vi "main.vi"() -> ()   [LabVIEW 2023] (continued)
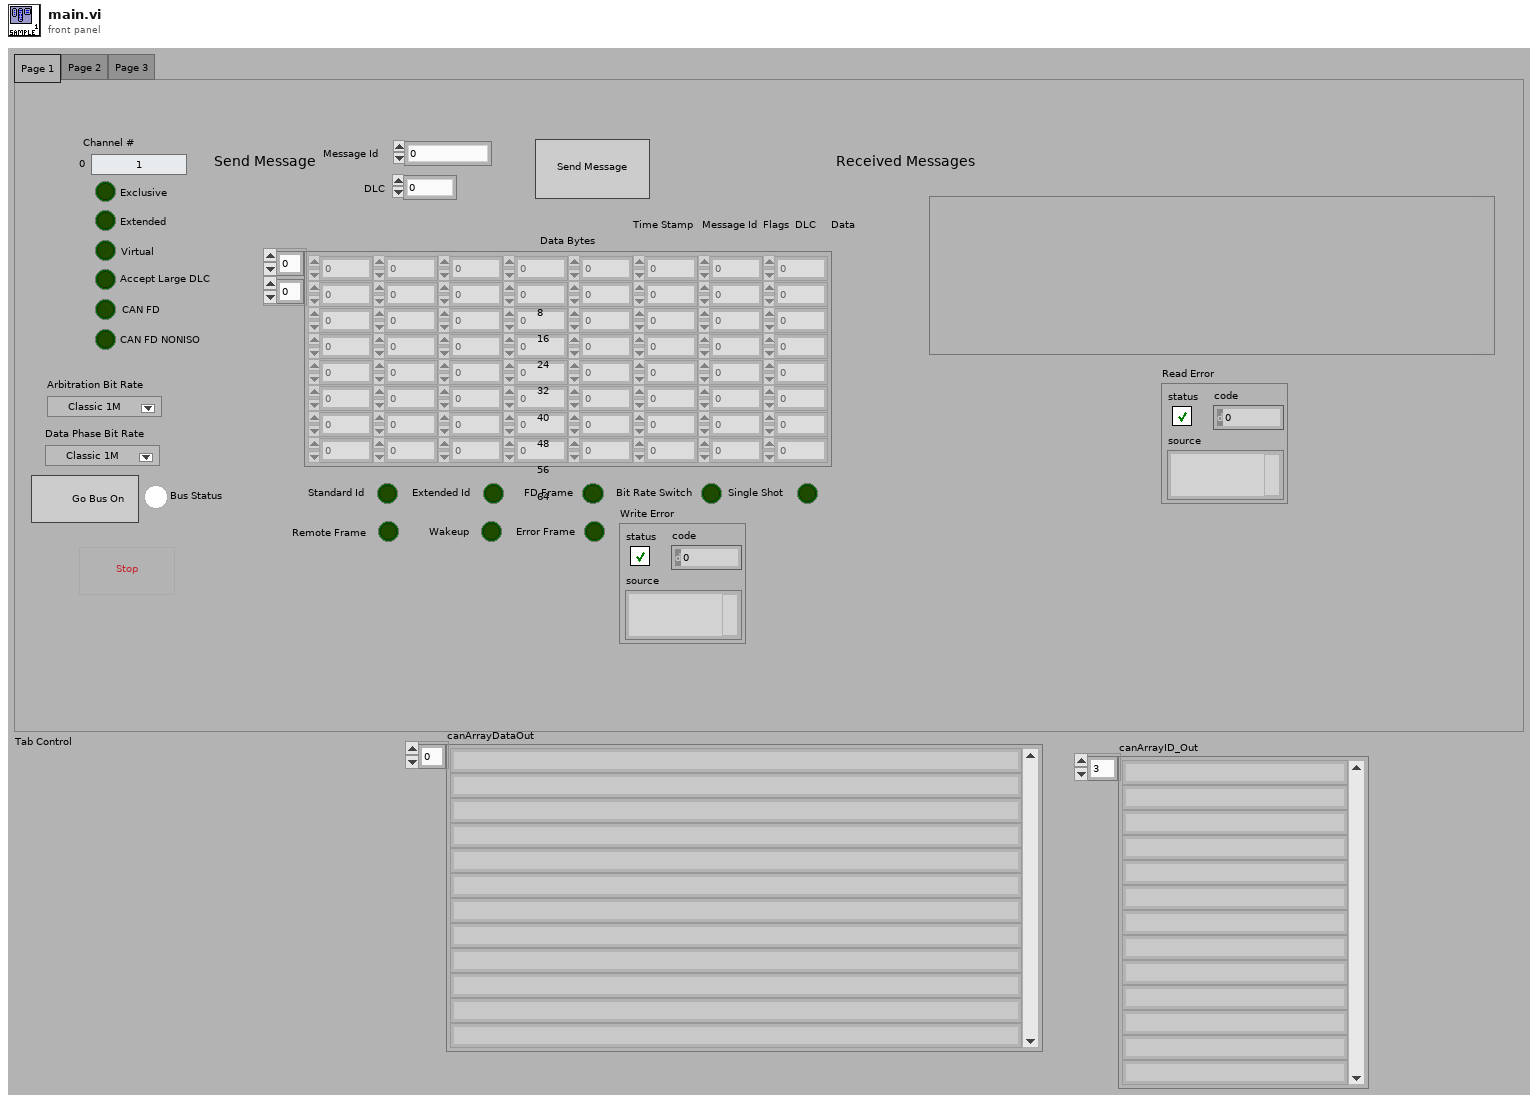
[diagram p1: front panel]
types:
  T1 = cluster{"flag 1":u32, "flag 2":u32, "flag 3":u32, "flag 4":u32}
  T2 = cluster{string, "Frame":refnum<k21>, "NameShort":string, "StartBit":u32, "NumBits":u32, "Min":dbl, "Max":dbl, "ScaleFac":dbl, "ScaleOff":dbl}[]
  T3 = typedef "readSub.ctl" = enum16{"Read", "Process"}
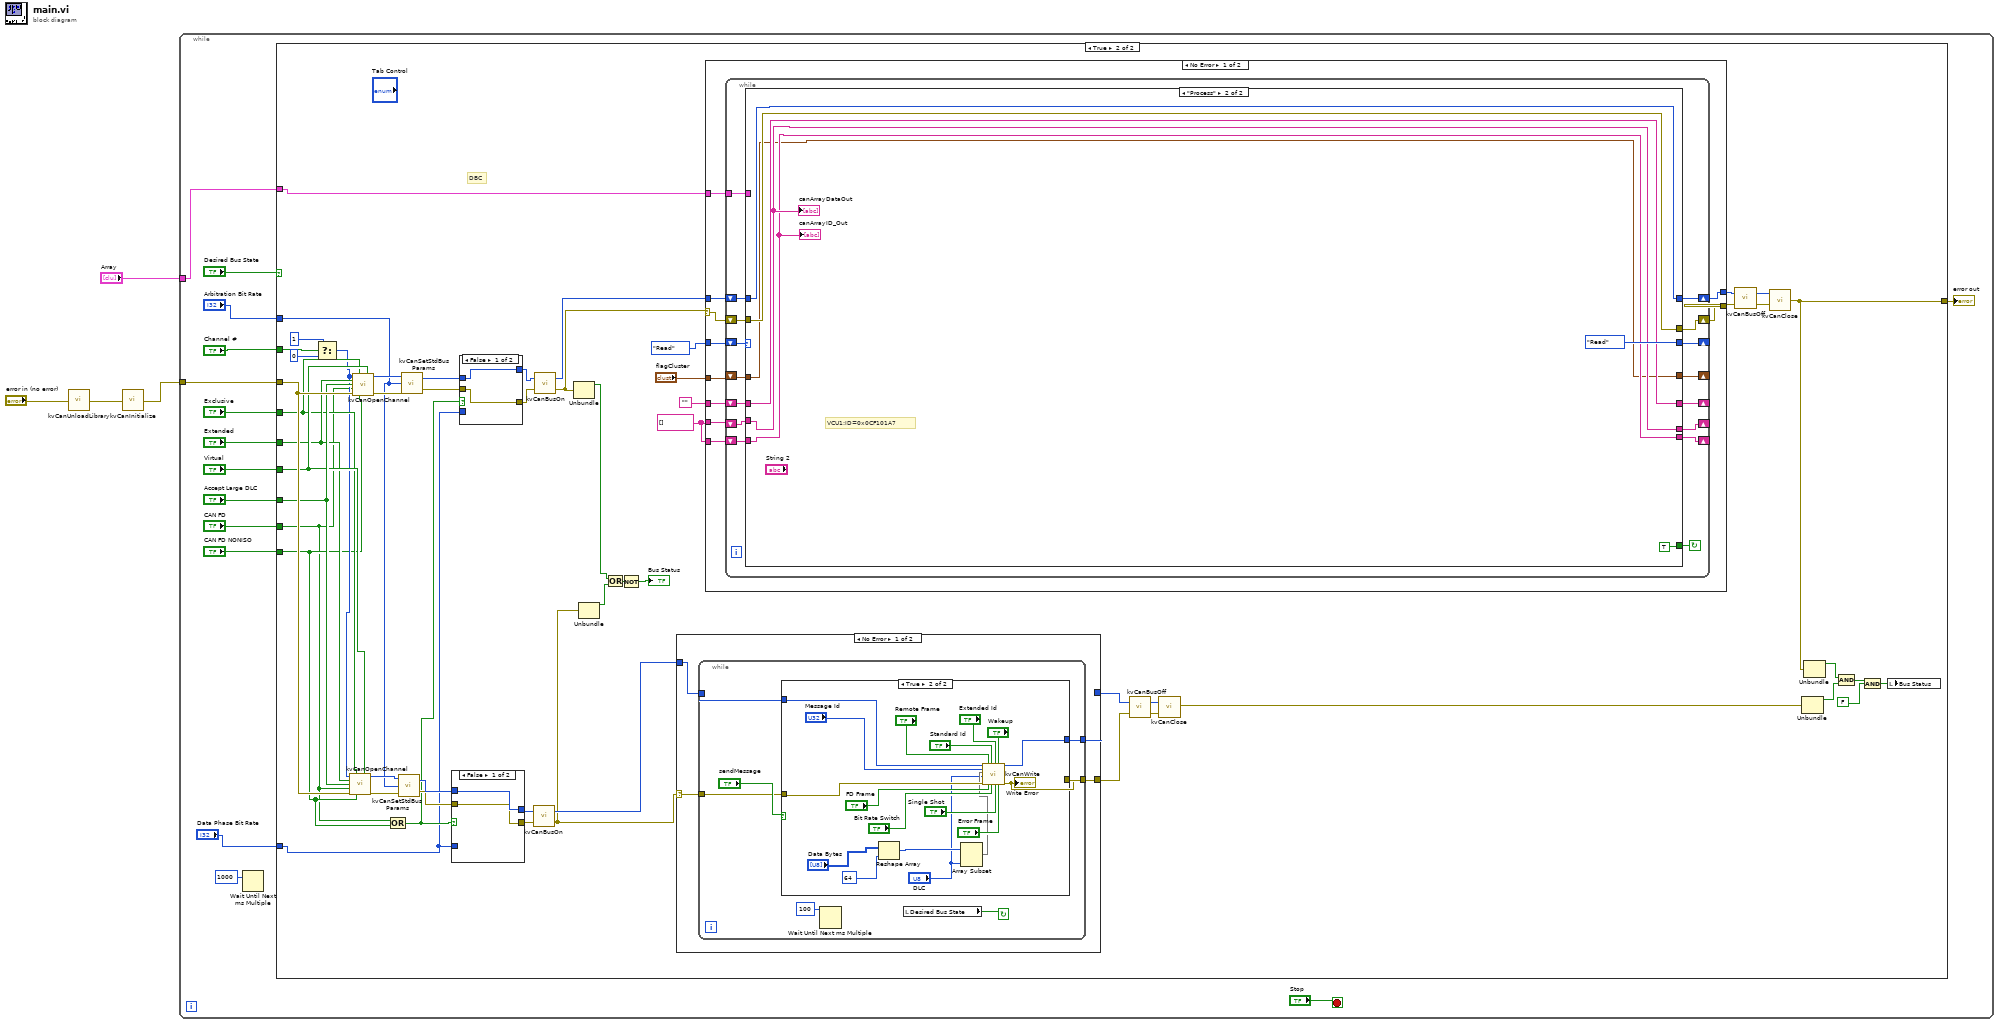
[diagram p0: block diagram]
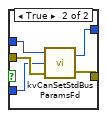
[diagram p3: hidden frame]
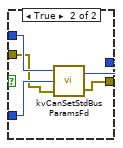
[diagram p6: hidden frame]
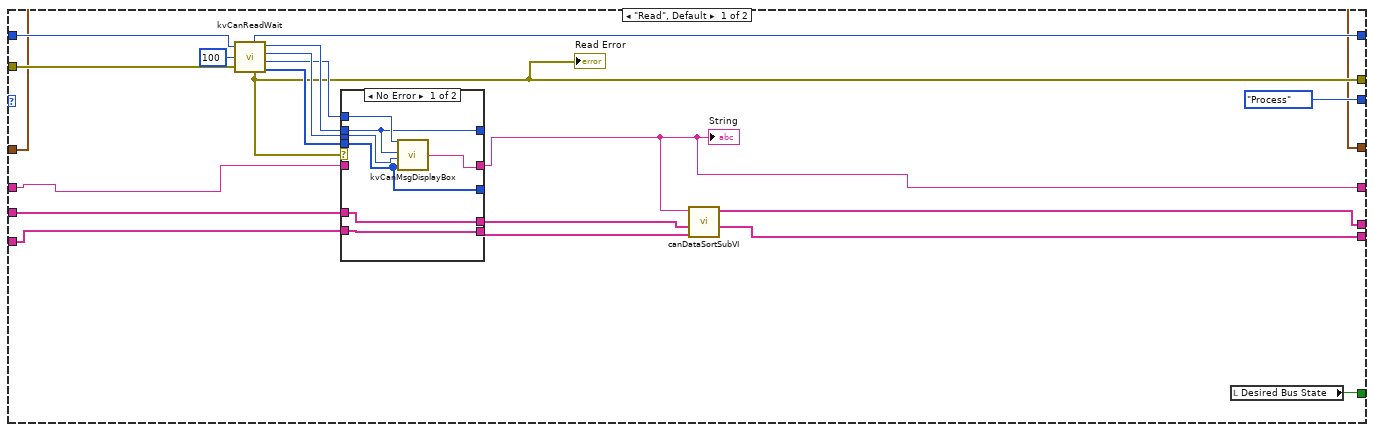
[diagram p7: hidden frame]
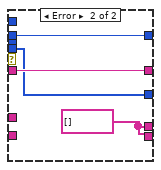
[diagram p8: hidden frame]
diagram:
  n1 = call "kvCanUnloadLibrary.vi"("error in (no error)"="error in (no error)") -> ("error out"=w3:errorcluster)
  n2 = call "kvCanInitialize.vi"("error in (no error)"=w3) -> ("error out (no error)"=w4:errorcluster)
  n3 = while {
    tunnel: w4 -> [w19]
    tunnel: "Array" -> [w5]
    stop <- "Stop" stop-if-true
    n4 = Wait Until Next ms Multiple(millisecond multiple=u32 1000) -> ()  [unwired: 1 out]
    n5 = case shown="True" "Desired Bus State" {
      tunnel: w19 -> [w20 w57]
      tunnel: "Arbitration Bit Rate" -> [_ w58]
      tunnel: "Channel #" -> [_ w61]
      tunnel: "Accept Large DLC" -> [_ w56]
      tunnel: "Extended" -> [_ w54]
      tunnel: "Virtual" -> [_ w55]
      tunnel: "Exclusive" -> [_ w53]
      tunnel: "CAN FD" -> [_ w50]
      tunnel: "CAN FD NONISO" -> [_ w51]
      tunnel: "Data Phase Bit Rate" -> [_ w27]
      tunnel: [w20 w26] -> w6
      tunnel: w5 -> [_ w23]
      frame False {
      }
      frame True {
        w22 = string[] [] ("appended array")
        # "DBC"
        n6 = Select(t=u32 1, s=w61, f=u32 0) -> (s? t:f=w52:u32)
        n7 = call "kvCanOpenChannel.vi"("CAN Channel Number"=w52, "WantExclusive"=w53, "AcceptVirtual"=w55, "WantExtended"=w54, "Accept Large DLC"=w56, "CAN FD"=w50, "error in (no error)"=w57, "CAN FD NONISO"=w51) -> ("Opened Channel Handle\n(output only)"=w59:i32, "error out"=w60:errorcluster)  [unwired: 6 in]
        n8 = call "kvCanOpenChannel.vi"("CAN Channel Number"=w52, "WantExclusive"=w53, "AcceptVirtual"=w55, "WantExtended"=w54, "Accept Large DLC"=w56, "CAN FD"=w50, "error in (no error)"=w57, "CAN FD NONISO"=w51) -> ("Opened Channel Handle\n(output only)"=w63:i32, "error out"=w62:errorcluster)  [unwired: 6 in]
        n9 = Or(x=w50, y=w51) -> (x .or. y?=w32:bool)
        n10 = call "kvCanSetStdBusParams.vi"("error in (no error)"=w60, "Standard CAN Baud Rate"=w58, "Channel Handle (input only)"=w59) -> ("error out"=w48:errorcluster, "Channel Handle (ouput only)"=w49:i32)
        n11 = call "kvCanSetStdBusParams.vi"("error in (no error)"=w62, "Standard CAN Baud Rate"=w58, "Channel Handle (input only)"=w63) -> ("error out"=w33:errorcluster, "Channel Handle (ouput only)"=w36:i32)
        n12 = case shown="False" w32 {
          tunnel: w49 -> [w116 w121]
          tunnel: w48 -> [w115 w119]
          tunnel: [w116 w117] -> w46
          tunnel: [w115 w118] -> w47
          tunnel: w27 -> [_ w120]
          frame False {
          }
          frame True {
            n13 = call "kvCanSetStdBusParamsFd.vi"("error in (no error)"=w119, "Standard CAN Baud Rate"=w120, "Channel Handle (input only)"=w121) -> ("error out"=w118:errorcluster, "Channel Handle (output only)"=w117:i32)
          }
        }
        n14 = case shown="False" w32 {
          tunnel: w36 -> [w76 w81]
          tunnel: [w76 w80] -> w35
          tunnel: [w75 w79] -> w34
          tunnel: w33 -> [w75 w78]
          tunnel: w27 -> [_ w77]
          frame False {
          }
          frame True {
            n15 = call "kvCanSetStdBusParamsFd.vi"("error in (no error)"=w78, "Standard CAN Baud Rate"=w77, "Channel Handle (input only)"=w81) -> ("error out"=w79:errorcluster, "Channel Handle (output only)"=w80:i32)
          }
        }
        n16 = call "kvCanBusOn.vi"("error in (no error)"=w47, "Channel Handle (input only)"=w46) -> ("error out"=w31:errorcluster, "Channel Handle (ouput only)"=w45:i32)
        n17 = call "kvCanBusOn.vi"("error in (no error)"=w34, "Channel Handle (input only)"=w35) -> ("error out"=w69:errorcluster, "Channel Handle (ouput only)"=w68:i32)
        n18 = Unbundle(w69) -> ("status"=w29:bool)  [unwired: 2 out]
        n19 = Unbundle(w31) -> ("status"=w30:bool)  [unwired: 2 out]
        n20 = Or(x=w29, y=w30) -> (x .or. y?=w28:bool)
        n21 = Not(x=w28) -> (.not. x?=→"Bus Status":bool)
        n22 = case shown="No Error" w31 {
          selector: w31 -> [w82 w114]
          tunnel: [w85 w114] -> w43
          tunnel: w45 -> [w84 w113]
          tunnel: [w83 w113] -> w44
          frame No Error {
            n23 = while {
              tunnel: [w89] -> w85
              tunnel: w84 -> [w88]
              tunnel: [w87] -> w83
              tunnel: w82 -> [w86]
              stop <- w90 continue-if-true
              n24 = case shown="True" "sendMessage" {
                tunnel: [w94 w112] -> w89
                tunnel: w88 -> [w93 w111]
                tunnel: [w93 w110] -> w87
                tunnel: w86 -> [w94 w109]
                frame False {
                }
                frame True {
                  n25 = Reshape Array("Data Bytes", 64 ("dimension size")) -> (w96:u8[])
                  n26 = Array Subset(array=w96, length="DLC") -> (w97:u8[])  [unwired: 1 in]
                  n27 = call "kvCanWrite.vi"("Channel Handle (input only)"=w111, "Message Id"="Message Id", "Message"=w97, "DLC"="DLC", "error in (no error)"=w109, "Remote Request"="Remote Frame", "FD Frame"="FD Frame", "Standard 11-bit Id"="Standard Id", "Bit Rate Switch"="Bit Rate Switch", "Extended 29-bit Id"="Extended Id", "Single Shot"="Single Shot", "Wakeup"="Wakeup", "Error Frame"="Error Frame") -> ("Channel Handle (output only)"=w110:i32, "error out"=w112:errorcluster)  [unwired: 5 in]
                  "Write Error" <- w112
                }
              }
              n28 = Wait Until Next ms Multiple(millisecond multiple=u32 100) -> ()  [unwired: 1 out]
              n29 = local read "Desired Bus State"() -> (w90:bool)
            }
          }
          frame Error {
          }
        }
        n30 = case shown="No Error" w69 {
          selector: w69 -> [w130 w188]
          tunnel: [w127 w188] -> w64
          tunnel: w68 -> [w131 w187]
          tunnel: [w129 w187] -> w65
          tunnel: "" -> [w128 _]
          tunnel: readSub."Read" -> [w126 _]
          tunnel: w23 -> [w125 _]
          tunnel: w22 -> [w124 _]
          tunnel: w22 -> [w123 _]
          tunnel: "flagCluster" -> [w122 _]
          frame No Error {
            n31 = while {
              shift-right: [w142] -> _
              shift-left: w128 -> [w143]
              shift-right: [w144] -> w129
              shift-left: w131 -> [w145]
              shift-right: [w141] -> w127
              shift-left: w130 -> [w146]
              shift-right: [w140] -> _
              shift-left: w126 -> [w139]
              tunnel: w125 -> [w138]
              shift-right: [w135] -> _
              shift-left: w124 -> [w137]
              shift-right: [w134] -> _
              shift-left: w123 -> [w136]
              shift-right: [w133] -> _
              shift-left: w122 -> [w132]
              stop <- w147 continue-if-true
              n32 = case shown="\"Process\"" w139 {
                tunnel: [w167 TRUE] -> w147
                tunnel: w146 -> [w162 w184]
                tunnel: w145 -> [w160 w185]
                tunnel: [w159 w185] -> w144
                tunnel: w143 -> [w156 w182]
                tunnel: [w151 w182] -> w142
                tunnel: [w158 w184] -> w141
                tunnel: [readSub."Process" readSub."Read"] -> w140
                tunnel: w138 -> [_ _]
                tunnel: w137 -> [w155 w181]
                tunnel: w136 -> [w154 w180]
                tunnel: [w150 w181] -> w135
                tunnel: [w149 w180] -> w134
                tunnel: [w148 w179] -> w133
                tunnel: w132 -> [w148 w179]
                frame "Read", Default {
                  n33 = call "kvCanReadWait.vi"("error in (no error)"=w162, "Read Timeout (ms)"=u32 100, "Channel Handle (input only)"=w160) -> ("Message Data"=w166:u8[], "error out"=w158:errorcluster, "Message Timestamp"=w163:u32, "Message Flags"=w165:u32, "Channel Handle (output only)"=w159:i32, "Message Id"=w164:i32)
                  "Read Error" <- w158
                  n34 = case shown="No Error" w158 {
                    tunnel: w156 -> [_ w178]
                    tunnel: [w174 w178] -> w151
                    tunnel: w166 -> [w169 w176]
                    tunnel: w165 -> [w173 _]
                    tunnel: w164 -> [w168 w175]
                    tunnel: w163 -> [w172 _]
                    tunnel: w155 -> [w171 _]
                    tunnel: w154 -> [w170 _]
                    tunnel: [w171 w177] -> w153
                    tunnel: [w170 w177] -> w152
                    tunnel: [w169 w176] -> _
                    tunnel: [w168 w175] -> _
                    frame No Error {
                      n35 = call "kvCanMsgDisplayBox.vi"("Message Data"=w169, "Message Flags"=w173, "Message Id"=w168, "Time Stamp"=w172) -> ("Output String"=w174:string)
                    }
                    frame Error {
                      w177 = string[] [] ("appended array")
                    }
                  }
                  "String" <- w151
                  n36 = call "canDataSortSubVI.vi"("canArrayID_In"=w152, "canArrayDataIn"=w153, "dataIn"=w151) -> ("canArrayID"=w149:string[], "canArrayData"=w150:string[])  [unwired: 7 in]
                  n37 = local read "Desired Bus State"() -> (w167:bool)
                }
                frame "Process" {
                  # "VCU1:ID=0x0CF101A7"
                  "canArrayDataOut" <- w181
                  "canArrayID_Out" <- w180
                }
              }
            }
          }
          frame Error {
          }
        }
        n38 = call "kvCanBusOff.vi"("error in (no error)"=w43, "Channel Handle (input only)"=w44) -> ("error out"=w42:errorcluster, "Channel Handle (ouput only)"=w41:i32)
        n39 = call "kvCanClose.vi"("error in (no error)"=w42, "Channel Handle (input only)"=w41) -> ("error out"=w40:errorcluster)
        n40 = call "kvCanBusOff.vi"("error in (no error)"=w64, "Channel Handle (input only)"=w65) -> ("error out"=w66:errorcluster, "Channel Handle (ouput only)"=w67:i32)
        n41 = call "kvCanClose.vi"("error in (no error)"=w66, "Channel Handle (input only)"=w67) -> ("error out"=w26:errorcluster)
        n42 = Unbundle(w40) -> ("status"=w38:bool)  [unwired: 2 out]
        n43 = Unbundle(w26) -> ("status"=w39:bool)  [unwired: 2 out]
        n44 = And(x=w39, y=w38) -> (x .and. y?=w37:bool)
        n45 = And(x=w37, y=FALSE) -> (x .and. y?=w71:bool)
        n46 = local write "Bus Status"(w71) -> ()
      }
    }
    "error out" <- w6
  }
